vi "Логи_GPS.vi"() -> ()   [LabVIEW 2013]
panel:
  in  "Tab Control":T1(tab)
  out "?":cluster{dbl[], dbl[]}[](graph)
  out "XY":cluster{dbl[], dbl[]}[](graph)
  out "speed":cluster{dbl[], dbl[]}[](graph)
  out "Координаты":cluster{dbl[], u32[]}[](graph)
  out "complementary":cluster{dbl[], dbl[]}[](graph)
  out "complementary 2":cluster{dbl[], dbl[]}[](graph)
  out "complementary 3":cluster{dbl[], dbl[]}[](graph)
  out "complementary 4":cluster{dbl[], dbl[]}[](graph)
  out "ID параметров":u8[](array[numeric])
  out "Длина заголовка":i32
  out "Заголовок":string
  out "Количество параметров":u8
  out "size (in bytes)":i64
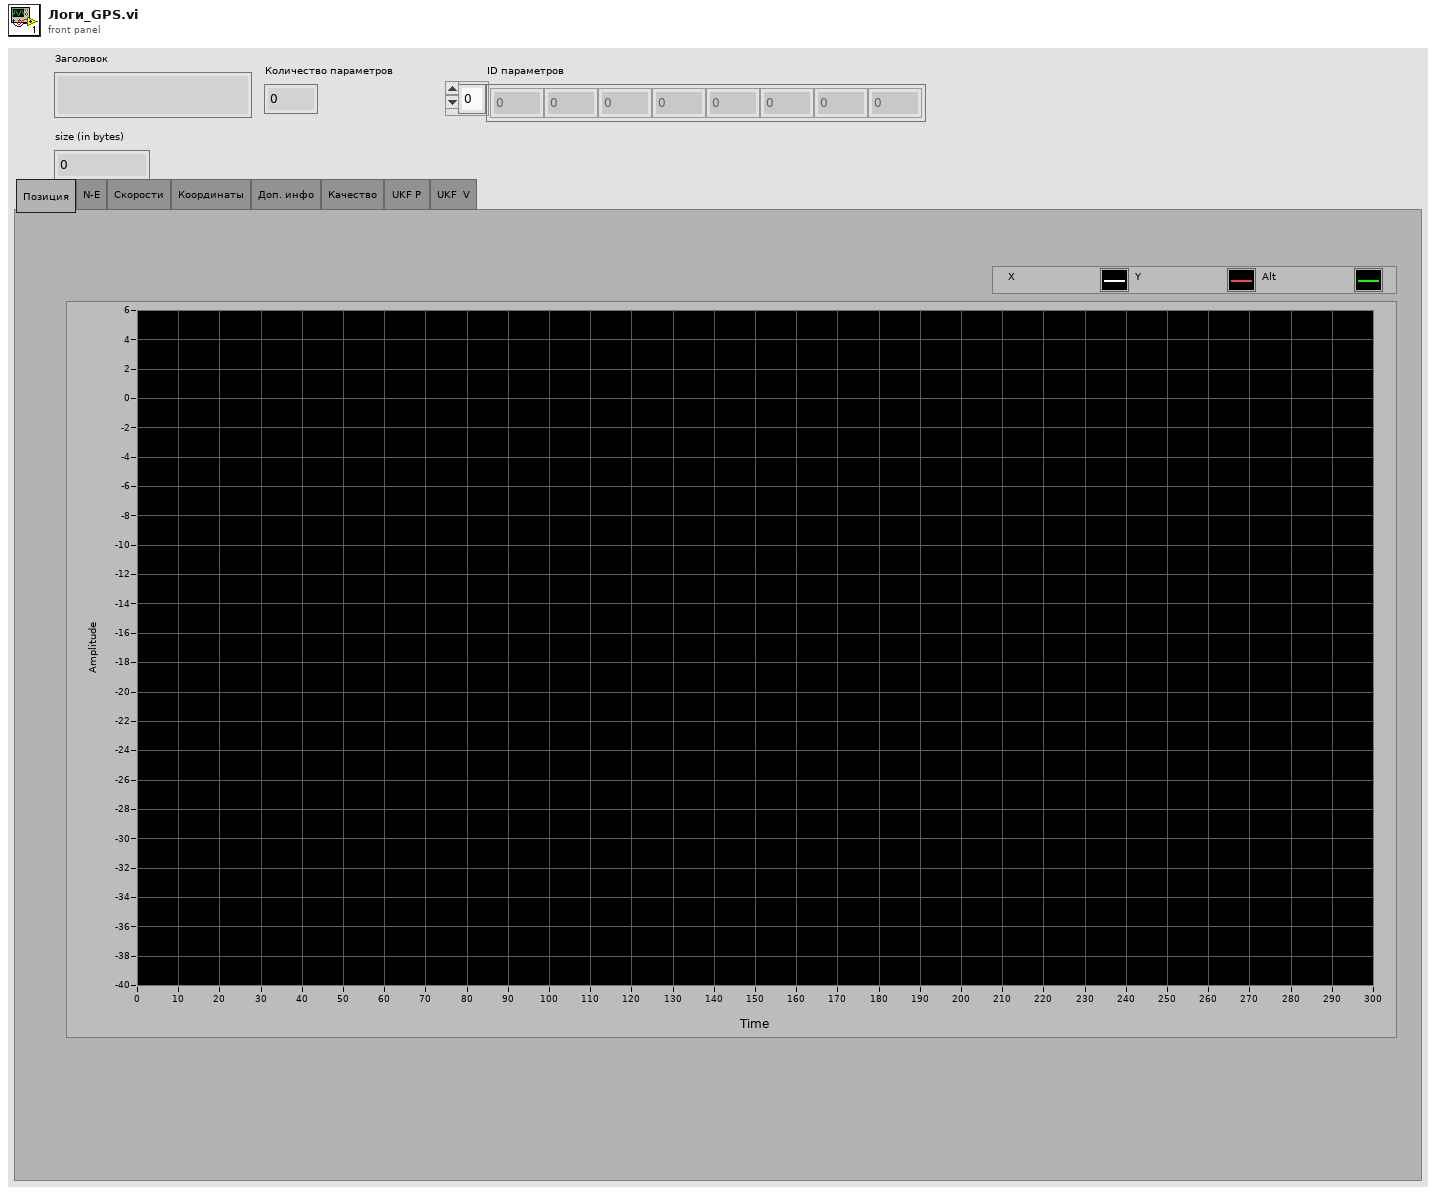
[diagram p1: front panel]
types:
  T1 = enum32{"Позиция", "N-E", "Скорости", "Координаты", "Доп. инфо", "Качество", "UKF P ", "UKF  V"}
  T2 = enum16{"open", "replace", "create", "open or create", "replace or create", "replace or create with confirmation"}
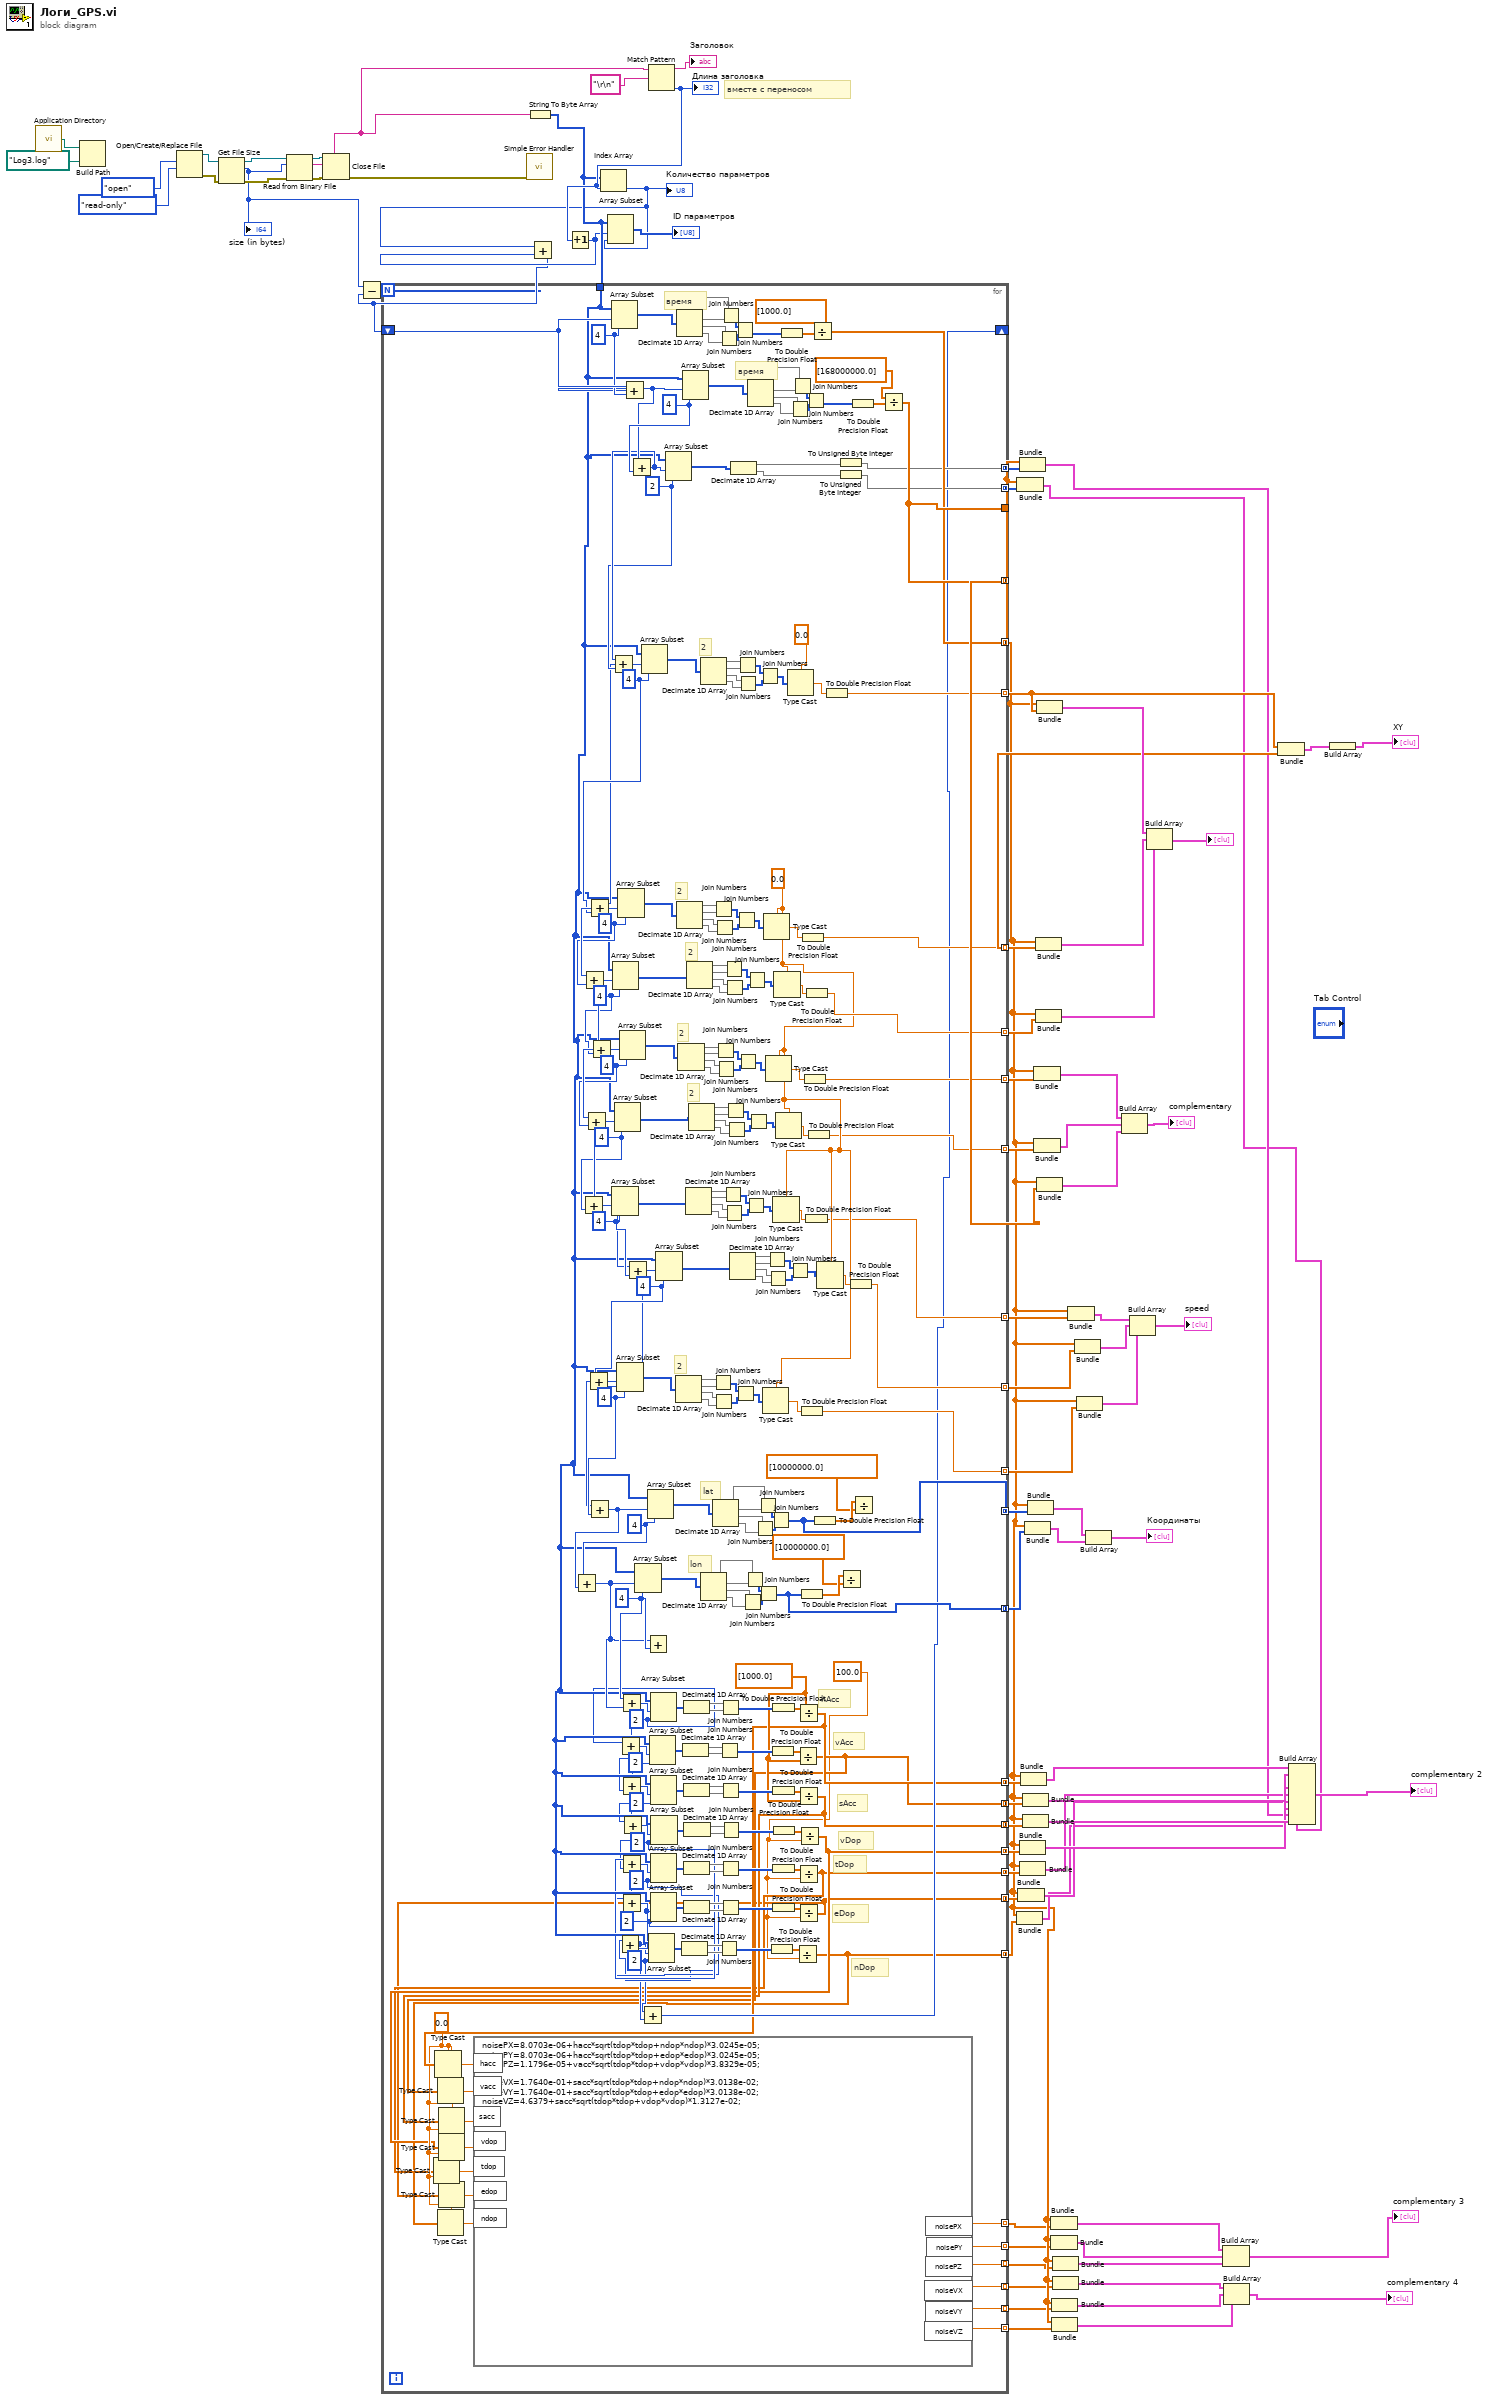
[diagram p0: block diagram]
diagram:
  # "вместе с переносом"
  n1 = call <vilib>:"Application Directory.vi"() -> ("Application Directory"=w81:path)
  n2 = Build Path(base path=w81, name or relative path=path "Log3.log" ("default name")) -> ()  [unwired: 1 out]
  n3 = Open/Create/Replace File(operation (0:open)=T2."open", access (0:read/write)=enum16{"read/write", "read-only", "write-only"}."read-only") -> (refnum out=w78:refnum<file>, error out=w76:errorcluster)  [unwired: 4 in, 1 out]
  n4 = Get File Size(file=w78, error in=w76) -> (refnum out=w77:refnum<file>, size (in bytes)=w68:i64, 0:w75:errorcluster)
  "size (in bytes)" <- w68
  n5 = Read from Binary File(8:w75, 10:w68, 11:w77) -> (0:w79:errorcluster, 2:w74:string, 3:w80:refnum<file>)  [unwired: 3 in, 1 out]
  n6 = Close File(refnum=w80, error in=w79) -> (error out=w84:errorcluster)  [unwired: 1 out]
  n7 = call <vilib>:"Simple Error Handler.vi"("error in (no error)"=w84) -> ()  [unwired: 4 in, 5 out]
  n8 = String To Byte Array(string=w74) -> (unsigned byte array=w69:u8[])
  n9 = Match Pattern(string=w74, regular expression="\r\n" ("format string")) -> (before substring=→"Заголовок":string, offset past match=w71:i32)  [unwired: 1 in, 2 out]
  "Длина заголовка" <- w71
  n10 = Increment(x=w71) -> (x+1=w66:i32)
  n11 = Index Array(array=w69, index=w71) -> (element=w67:u8)
  "Количество параметров" <- w67
  n12 = Add(x=w67, y=w66) -> (x+y=w65:i32)
  n13 = Subtract(x=w68, y=w65) -> (x-y=w64:i64)
  n14 = for {
    N: w64 -> [_]
    tunnel: w69 -> [w130]
    shift-right: [w115] -> _
    shift-left: w65 -> [w295]
    tunnel: [w291] -> w33 mode=concatenating
    tunnel: [w291] -> _
    tunnel: [w270] -> w46 mode=indexing
    tunnel: [w269] -> w48 mode=indexing
    tunnel: [w167] -> w61 mode=indexing
    tunnel: [w166] -> w60 mode=indexing
    tunnel: [w235] -> w15 mode=concatenating
    tunnel: [w230] -> w58 mode=concatenating
    tunnel: [w229] -> w57 mode=concatenating
    tunnel: [w213] -> w47 mode=indexing
    tunnel: [w183] -> w43 mode=concatenating
    tunnel: [w182] -> w42 mode=concatenating
    tunnel: [w165] -> w40 mode=indexing
    tunnel: [w164] -> w39 mode=indexing
    tunnel: [w163] -> w38 mode=indexing
    tunnel: [w100] -> w24 mode=concatenating
    tunnel: [w96] -> w23 mode=concatenating
    tunnel: [w95] -> w22 mode=concatenating
    tunnel: [w94] -> w21 mode=concatenating
    tunnel: [w93] -> w20 mode=concatenating
    tunnel: [w92] -> w19 mode=concatenating
    tunnel: [w91] -> w18 mode=concatenating
    tunnel: [w106] -> w14 mode=indexing
    tunnel: [w105] -> w13 mode=indexing
    tunnel: [w104] -> w12 mode=indexing
    tunnel: [w103] -> w11 mode=indexing
    tunnel: [w102] -> w10 mode=indexing
    tunnel: [w101] -> w9 mode=indexing
    w85 = 100.0
    w98 = sgl 0.0
    w107 = dbl[] [1000.0] ("y")
    w117 = 2 ("length")
    w119 = 2 ("length")
    w121 = 2 ("length")
    w123 = 2 ("length")
    w125 = 2 ("length")
    w127 = 2 ("length")
    w129 = 2 ("length")
    w172 = 4 ("length")
    w156 = 4 ("length")
    w189 = 4 ("length")
    w162 = 4 ("length")
    w217 = 4 ("length")
    w215 = 2 ("length")
    w170 = 4 ("length")
    w236 = 4 ("length")
    w267 = 4 ("length")
    w168 = sgl 0.0
    w247 = 4 ("length")
    w289 = 4 ("length")
    w231 = 4 ("length")
    w294 = 4 ("length")
    # "nDop"
    # "eDop"
    # "tDop"
    # "vDop"
    # "sAcc"
    # "vAcc"
    # "hAcc"
    # "lon"
    # "lat"
    # "2"
    # "2"
    # "2"
    # "2"
    # "2"
    # "2"
    # "время"
    # "время"
    n15 = Array Subset(array=w130, index=w295, length=w294) -> (w307:u8[])
    n16 = Add(x=w295, y=w294) -> (x+y=w228:i32)
    n17 = Add(x=w228, y=w231) -> (x+y=w216:i32)
    n18 = Add(x=w216, y=w215) -> (x+y=w214:i32)
    n19 = Add(x=w214, y=w217) -> (x+y=w290:i32)
    n20 = Add(x=w290, y=w289) -> (x+y=w248:i32)
    n21 = Add(x=w248, y=w247) -> (x+y=w268:i32)
    n22 = Add(x=w268, y=w267) -> (x+y=w237:i32)
    n23 = Add(x=w237, y=w236) -> (x+y=w169:i32)
    n24 = Array Subset(array=w130, index=w169, length=w170) -> (w240:u8[])
    n25 = Array Subset(array=w130, index=w248, length=w247) -> (w275:u8[])
    n26 = Array Subset(array=w130, index=w237, length=w236) -> (w253:u8[])
    n27 = Array Subset(array=w130, index=w290, length=w289) -> (w286:u8[])
    n28 = Array Subset(array=w130, index=w268, length=w267) -> (w264:u8[])
    n29 = Add(x=w169, y=w170) -> (x+y=w171:i32)
    n30 = Add(x=w172, y=w171) -> (x+y=w161:i32)
    n31 = Add(x=w161, y=w162) -> (x+y=w188:i32)
    n32 = Add(x=w189, y=w188) -> (x+y=w155:i32)
    n33 = Array Subset(array=w130, index=w161, length=w162) -> (w210:u8[])
    n34 = Add(x=w156, y=w155) -> (x+y=w128:i32)
    n35 = Add(x=w129, y=w128) -> (x+y=w126:i32)
    n36 = Add(x=w127, y=w126) -> (x+y=w124:i32)
    n37 = Add(x=w125, y=w124) -> (x+y=w122:i32)
    n38 = Add(x=w123, y=w122) -> (x+y=w120:i32)
    n39 = Add(x=w121, y=w120) -> (x+y=w118:i32)
    n40 = Add(x=w119, y=w118) -> (x+y=w116:i32)
    n41 = Array Subset(array=w130, index=w155, length=w156) -> (w190:u8[])
    n42 = Add(x=w117, y=w116) -> (x+y=w115:i32)
    n43 = Array Subset(array=w130, index=w214, length=w217) -> (w225:u8[])
    n44 = Add(x=w155, y=w156) -> ()  [unwired: 1 out]
    n45 = Array Subset(array=w130, index=w188, length=w189) -> (w197:u8[])
    n46 = Array Subset(array=w130, index=w116, length=w117) -> (w132:u8[])
    n47 = Array Subset(array=w130, index=w126, length=w127) -> (w152:u8[])
    n48 = Array Subset(array=w130, index=w128, length=w129) -> (w158:u8[])
    n49 = Array Subset(array=w130, index=w124, length=w125) -> (w148:u8[])
    n50 = Array Subset(array=w130, index=w120, length=w121) -> (w140:u8[])
    n51 = Array Subset(array=w130, index=w118, length=w119) -> (w136:u8[])
    n52 = Array Subset(array=w130, index=w122, length=w123) -> (w144:u8[])
    n53 = Array Subset(array=w130, index=w171, length=w172) -> (w175:u8[])
    n54 = Array Subset(array=w130, index=w216, length=w215) -> (w234:u8[])
    n55 = Decimate 1D Array(w210) -> (w211:u8[], w212:u8[], w209:u8[], w208:u8[])
    n56 = Decimate 1D Array(w307) -> (w309:u8[], w310:u8[], w311:u8[], w312:u8[])
    n57 = Decimate 1D Array(w286) -> (w287:u8[], w288:u8[], w285:u8[], w284:u8[])
    n58 = Decimate 1D Array(w264) -> (w265:u8[], w266:u8[], w263:u8[], w262:u8[])
    n59 = Decimate 1D Array(w132) -> (w133:u8[], w134:u8[])
    n60 = Array Subset(array=w130, index=w228, length=w231) -> (w297:u8[])
    n61 = Decimate 1D Array(w152) -> (w153:u8[], w154:u8[])
    n62 = Decimate 1D Array(w158) -> (w159:u8[], w160:u8[])
    n63 = Decimate 1D Array(w148) -> (w149:u8[], w150:u8[])
    n64 = Decimate 1D Array(w140) -> (w141:u8[], w142:u8[])
    n65 = Decimate 1D Array(w136) -> (w137:u8[], w138:u8[])
    n66 = Decimate 1D Array(w144) -> (w145:u8[], w146:u8[])
    n67 = Decimate 1D Array(w240) -> (w245:u8[], w246:u8[], w244:u8[], w243:u8[])
    n68 = Decimate 1D Array(w275) -> (w280:u8[], w281:u8[], w279:u8[], w278:u8[])
    n69 = Decimate 1D Array(w253) -> (w258:u8[], w259:u8[], w257:u8[], w256:u8[])
    n70 = Decimate 1D Array(w225) -> (w226:u8[], w227:u8[], w224:u8[], w223:u8[])
    n71 = Decimate 1D Array(w190) -> (w192:u8[], w193:u8[], w194:u8[], w195:u8[])
    n72 = Join Numbers(hi=w211, lo=w212) -> ((hi.lo)=w207:u16[])
    n73 = Join Numbers(hi=w287, lo=w288) -> ((hi.lo)=w283:u16[])
    n74 = Join Numbers(hi=w209, lo=w208) -> ((hi.lo)=w206:u16[])
    n75 = Join Numbers(hi=w285, lo=w284) -> ((hi.lo)=w282:u16[])
    n76 = Join Numbers(hi=w265, lo=w266) -> ((hi.lo)=w261:u16[])
    n77 = Decimate 1D Array(w197) -> (w199:u8[], w200:u8[], w201:u8[], w202:u8[])
    n78 = Join Numbers(hi=w263, lo=w262) -> ((hi.lo)=w260:u16[])
    n79 = Join Numbers(hi=w311, lo=w312) -> ((hi.lo)=w308:u16[])
    n80 = Join Numbers(hi=w133, lo=w134) -> ((hi.lo)=w108:u16[])
    n81 = Join Numbers(hi=w153, lo=w154) -> ((hi.lo)=w113:u16[])
    n82 = Join Numbers(hi=w159, lo=w160) -> ((hi.lo)=w114:u16[])
    n83 = Join Numbers(hi=w149, lo=w150) -> ((hi.lo)=w112:u16[])
    n84 = Join Numbers(hi=w141, lo=w142) -> ((hi.lo)=w110:u16[])
    n85 = Join Numbers(hi=w137, lo=w138) -> ((hi.lo)=w109:u16[])
    n86 = Join Numbers(hi=w309, lo=w310) -> ((hi.lo)=w313:u16[])
    n87 = Join Numbers(hi=w145, lo=w146) -> ((hi.lo)=w111:u16[])
    n88 = Join Numbers(hi=w245, lo=w246) -> ((hi.lo)=w242:u16[])
    n89 = Join Numbers(hi=w280, lo=w281) -> ((hi.lo)=w277:u16[])
    n90 = Join Numbers(hi=w244, lo=w243) -> ((hi.lo)=w241:u16[])
    n91 = Join Numbers(hi=w279, lo=w278) -> ((hi.lo)=w276:u16[])
    n92 = Join Numbers(hi=w258, lo=w259) -> ((hi.lo)=w255:u16[])
    n93 = Join Numbers(hi=w257, lo=w256) -> ((hi.lo)=w254:u16[])
    n94 = Decimate 1D Array(w175) -> (w180:u8[], w181:u8[], w179:u8[], w178:u8[])
    n95 = Decimate 1D Array(w234) -> (w233:u8[], w232:u8[])
    n96 = Join Numbers(hi=w313, lo=w308) -> ((hi.lo)=w304:u32[])
    n97 = Join Numbers(hi=w207, lo=w206) -> ((hi.lo)=w205:u32[])
    n98 = Join Numbers(hi=w283, lo=w282) -> ((hi.lo)=w272:u32[])
    n99 = Join Numbers(hi=w226, lo=w227) -> ((hi.lo)=w222:u16[])
    n100 = Join Numbers(hi=w224, lo=w223) -> ((hi.lo)=w221:u16[])
    n101 = Join Numbers(hi=w261, lo=w260) -> ((hi.lo)=w250:u32[])
    n102 = Join Numbers(hi=w194, lo=w195) -> ((hi.lo)=w191:u16[])
    n103 = Join Numbers(hi=w192, lo=w193) -> ((hi.lo)=w196:u16[])
    n104 = Join Numbers(hi=w242, lo=w241) -> ((hi.lo)=w239:u32[])
    n105 = Join Numbers(hi=w277, lo=w276) -> ((hi.lo)=w274:u32[])
    n106 = Join Numbers(hi=w255, lo=w254) -> ((hi.lo)=w252:u32[])
    n107 = Decimate 1D Array(w297) -> (w299:u8[], w300:u8[], w301:u8[], w302:u8[])
    n108 = Join Numbers(hi=w201, lo=w202) -> ((hi.lo)=w198:u16[])
    n109 = Join Numbers(hi=w199, lo=w200) -> ((hi.lo)=w203:u16[])
    n110 = Join Numbers(hi=w196, lo=w191) -> ((hi.lo)=w182:u32[])
    n111 = Join Numbers(hi=w222, lo=w221) -> ((hi.lo)=w220:u32[])
    n112 = Type Cast(type=w168, x=w205) -> (*(type *) &x=w204:sgl)
    n113 = Type Cast(type=w168, x=w272) -> (*(type *) &x=w271:sgl)
    n114 = Join Numbers(hi=w180, lo=w181) -> ((hi.lo)=w177:u16[])
    n115 = Type Cast(type=w168, x=w250) -> (*(type *) &x=w249:sgl)
    n116 = Join Numbers(hi=w179, lo=w178) -> ((hi.lo)=w176:u16[])
    n117 = Join Numbers(hi=w203, lo=w198) -> ((hi.lo)=w183:u32[])
    n118 = To Double Precision Float(number=w108) -> (double precision float=w131:dbl[])
    n119 = To Double Precision Float(number=w113) -> (double precision float=w151:dbl[])
    n120 = To Double Precision Float(number=w114) -> (double precision float=w157:dbl[])
    n121 = To Double Precision Float(number=w112) -> (double precision float=w147:dbl[])
    n122 = To Double Precision Float(number=w110) -> (double precision float=w139:dbl[])
    n123 = To Double Precision Float(number=w109) -> (double precision float=w135:dbl[])
    n124 = To Double Precision Float(number=w111) -> (double precision float=w143:dbl[])
    n125 = Type Cast(type=w168, x=w239) -> (*(type *) &x=w238:sgl)
    n126 = Type Cast(type=w168, x=w274) -> (*(type *) &x=w273:sgl)
    n127 = Type Cast(type=w168, x=w252) -> (*(type *) &x=w251:sgl)
    n128 = To Double Precision Float(number=w304) -> (double precision float=w306:dbl[])
    n129 = Join Numbers(hi=w301, lo=w302) -> ((hi.lo)=w298:u16[])
    n130 = Type Cast(type=sgl 0.0, x=w220) -> (*(type *) &x=w219:sgl)
    n131 = Join Numbers(hi=w177, lo=w176) -> ((hi.lo)=w174:u32[])
    n132 = Join Numbers(hi=w299, lo=w300) -> ((hi.lo)=w303:u16[])
    n133 = Divide(x=w131, y=w85) -> (x/y=w91:dbl[])
    n134 = Type Cast(type=w98, x=w91) -> (*(type *) &x=w86:sgl)
    n135 = Divide(x=w151, y=w107) -> (x/y=w96:dbl[])
    n136 = Type Cast(type=w98, x=w96) -> (*(type *) &x=w97:sgl)
    n137 = Divide(x=w157, y=w107) -> (x/y=w100:dbl[])
    n138 = Type Cast(type=w98, x=w100) -> (*(type *) &x=w99:sgl)
    n139 = Divide(x=w147, y=w107) -> (x/y=w95:dbl[])
    n140 = Type Cast(type=w98, x=w95) -> (*(type *) &x=w90:sgl)
    n141 = Divide(x=w139, y=w85) -> (x/y=w93:dbl[])
    n142 = Type Cast(type=w98, x=w93) -> (*(type *) &x=w88:sgl)
    n143 = Divide(x=w135, y=w85) -> (x/y=w92:dbl[])
    n144 = Type Cast(type=w98, x=w92) -> (*(type *) &x=w87:sgl)
    n145 = Divide(x=w143, y=w85) -> (x/y=w94:dbl[])
    n146 = Type Cast(type=w98, x=w94) -> (*(type *) &x=w89:sgl)
    n147 = formula code="noisePX=8.0703e-06+hacc*sqrt(tdop*tdop+ndop*ndop)*3.0245e-05;\nnoisePY=8.0703e-06+hacc*sqrt(tdop*tdop+edop*edop)*3.0245e-05;\nnoisePZ=1.1796e-05+vacc*sqrt(tdop*tdop+vdop*vdop)*3.8329e-05;\n\nnoiseVX=1.7640e-01+sacc*sqrt(tdop*tdop+ndop*ndop)*3.0138e-02;\nnoiseVY=1.7640e-01+sacc*sqrt(tdop*tdop+edop*edop)*3.0138e-02;\nnoiseVZ=4.6379+sacc*sqrt(tdop*tdop+vdop*vdop)*1.3127e-02;"("hacc"=w99, "vacc"=w97, "sacc"=w90, "vdop"=w89, "tdop"=w88, "edop"=w87, "ndop"=w86) -> ("noisePX"=w106:dbl, "noisePY"=w105:dbl, "noisePZ"=w104:dbl, "noiseVX"=w103:dbl, "noiseVY"=w102:dbl, "noiseVZ"=w101:dbl)
    n148 = To Double Precision Float(number=w204) -> (double precision float=w163:dbl)
    n149 = To Double Precision Float(number=w182) -> (double precision float=w185:dbl[])
    n150 = To Double Precision Float(number=w271) -> (double precision float=w270:dbl)
    n151 = To Double Precision Float(number=w249) -> (double precision float=w167:dbl)
    n152 = Join Numbers(hi=w303, lo=w298) -> ((hi.lo)=w296:u32[])
    n153 = To Double Precision Float(number=w238) -> (double precision float=w165:dbl)
    n154 = To Double Precision Float(number=w273) -> (double precision float=w269:dbl)
    n155 = To Double Precision Float(number=w251) -> (double precision float=w166:dbl)
    n156 = Divide(x=w306, y=dbl[] [1000.0]) -> (x/y=w235:dbl[])
    n157 = To Double Precision Float(number=w183) -> (double precision float=w187:dbl[])
    n158 = Type Cast(type=w168, x=w174) -> (*(type *) &x=w173:sgl)
    n159 = To Double Precision Float(number=w219) -> (double precision float=w213:dbl)
    n160 = To Unsigned Byte Integer(number=w233) -> (unsigned 8bit integer=w230:u8[])
    n161 = To Unsigned Byte Integer(number=w232) -> (unsigned 8bit integer=w229:u8[])
    n162 = Divide(x=w185, y=dbl[] [10000000.0]) -> ()  [unwired: 1 out]
    n163 = To Double Precision Float(number=w173) -> (double precision float=w164:dbl)
    n164 = To Double Precision Float(number=w296) -> (double precision float=w293:dbl[])
    n165 = Divide(x=w187, y=dbl[] [10000000.0]) -> ()  [unwired: 1 out]
    n166 = Divide(x=dbl[] [168000000.0] ("y"), y=w293) -> (x/y=w291:dbl[])
  }
  n167 = Array Subset(array=w69, index=w66, length=w67) -> (→"ID параметров":u8[])
  n168 = Bundle(w15, w18) -> (w25:cluster{dbl[], dbl[]})  [unwired: 1 in]
  n169 = Bundle(w15, w57) -> (w16:cluster{dbl[], u8[]})  [unwired: 1 in]
  n170 = Bundle(w15, w19) -> (w26:cluster{dbl[], dbl[]})  [unwired: 1 in]
  n171 = Bundle(w15, w58) -> (w17:cluster{dbl[], u8[]})  [unwired: 1 in]
  n172 = Bundle(w15, w21) -> (w28:cluster{dbl[], dbl[]})  [unwired: 1 in]
  n173 = Bundle(w15, w20) -> (w27:cluster{dbl[], dbl[]})  [unwired: 1 in]
  n174 = Bundle(w15, w24) -> (w32:cluster{dbl[], dbl[]})  [unwired: 1 in]
  n175 = Bundle(w15, w23) -> (w31:cluster{dbl[], dbl[]})  [unwired: 1 in]
  n176 = Bundle(w15, w22) -> (w30:cluster{dbl[], dbl[]})  [unwired: 1 in]
  n177 = Bundle(w15, w42) -> (w44:cluster{dbl[], u32[]})  [unwired: 1 in]
  n178 = Bundle(w15, w43) -> (w45:cluster{dbl[], u32[]})  [unwired: 1 in]
  n179 = Bundle(w15, w61) -> (w53:cluster{dbl[], dbl[]})  [unwired: 1 in]
  n180 = Bundle(w15, w60) -> (w52:cluster{dbl[], dbl[]})  [unwired: 1 in]
  n181 = Bundle(w15, w46) -> (w55:cluster{dbl[], dbl[]})  [unwired: 1 in]
  n182 = Bundle(w15, w48) -> (w54:cluster{dbl[], dbl[]})  [unwired: 1 in]
  n183 = Bundle(w15, w47) -> (w56:cluster{dbl[], dbl[]})  [unwired: 1 in]
  n184 = Bundle(w15, w33) -> (w51:cluster{dbl[], dbl[]})  [unwired: 1 in]
  n185 = Bundle(w15, w14) -> (w8:cluster{dbl[], dbl[]})  [unwired: 1 in]
  n186 = Bundle(w15, w13) -> (w7:cluster{dbl[], dbl[]})  [unwired: 1 in]
  n187 = Bundle(w15, w10) -> (w2:cluster{dbl[], dbl[]})  [unwired: 1 in]
  n188 = Bundle(w15, w9) -> (w1:cluster{dbl[], dbl[]})  [unwired: 1 in]
  n189 = Bundle(w15, w12) -> (w6:cluster{dbl[], dbl[]})  [unwired: 1 in]
  n190 = Bundle(w15, w11) -> (w3:cluster{dbl[], dbl[]})  [unwired: 1 in]
  n191 = Bundle(w15, w40) -> (w37:cluster{dbl[], dbl[]})  [unwired: 1 in]
  n192 = Bundle(w15, w39) -> (w36:cluster{dbl[], dbl[]})  [unwired: 1 in]
  n193 = Bundle(w15, w38) -> (w35:cluster{dbl[], dbl[]})  [unwired: 1 in]
  n194 = Build Array(w45, w44) -> (→"Координаты":cluster{dbl[], u32[]}[])
  n195 = Build Array(w53, w52, w51) -> (→"complementary":cluster{dbl[], dbl[]}[])
  n196 = Build Array(w37, w36, w35) -> (→"speed":cluster{dbl[], dbl[]}[])
  n197 = Build Array(w56, w55, w54) -> (→"?":cluster{dbl[], dbl[]}[])
  n198 = Build Array(w8, w7, w6) -> (→"complementary 3":cluster{dbl[], dbl[]}[])
  n199 = Build Array(w3, w2, w1) -> (→"complementary 4":cluster{dbl[], dbl[]}[])
  n200 = Bundle(w47, w46) -> (w50:cluster{dbl[], dbl[]})  [unwired: 1 in]
  n201 = Build Array(w32, w31, w30, w28, w27, w26, w25, w17, w16) -> (→"complementary 2":cluster{dbl[], dbl[]}[])
  n202 = Build Array(w50) -> (→"XY":cluster{dbl[], dbl[]}[])
